vi "HW5p1_Task1_Solution (2).vi"() -> ()   [LabVIEW 2016]
panel:
  out "D (nC/cm^2)":dbl
  in  "r (cm)":dbl
  in  "rho_v (nC/cm^3)":dbl
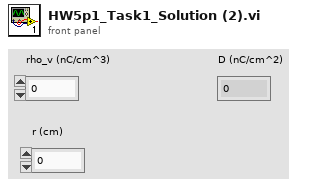
[diagram p1: front panel]
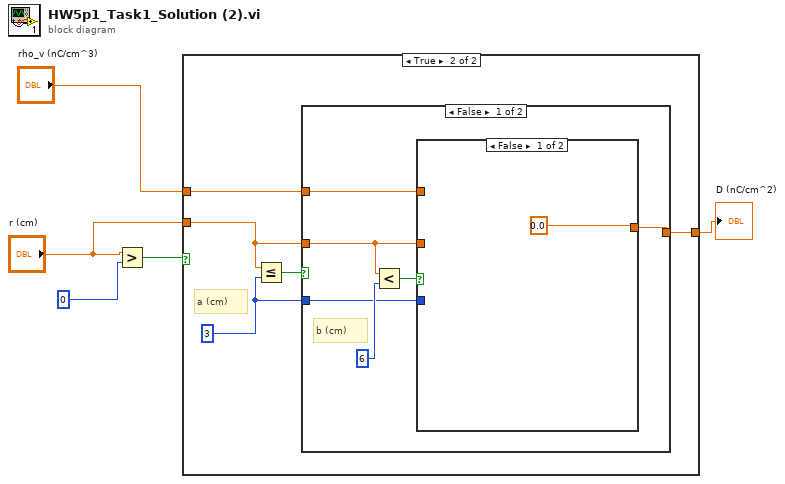
[diagram p0: block diagram]
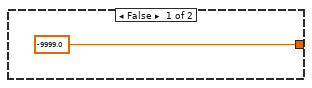
[diagram p2: hidden frame]
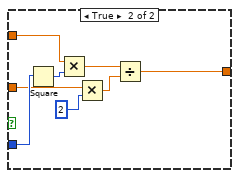
[diagram p3: hidden frame]
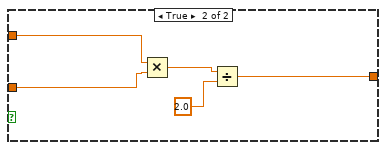
[diagram p4: hidden frame]
diagram:
  n1 = Greater?(x="r (cm)", y=0) -> (0:w5:bool)
  n2 = case shown="True" w5 {
    tunnel: "r (cm)" -> [_ w9]
    tunnel: "rho_v (nC/cm^3)" -> [_ w10]
    tunnel: [-9999.0 w8] -> w1
    frame False {
    }
    frame True {
      w7 = 3
      # "a (cm)"
      n3 = Less Or Equal?(x=w9, y=w7) -> (x <= y?=w11:bool)
      n4 = case shown="False" w11 {
        tunnel: w10 -> [w15 w31]
        tunnel: w9 -> [w13 w30]
        tunnel: [w12 w27] -> w8
        tunnel: w7 -> [w14 _]
        frame False {
          # "b (cm)"
          n5 = Less?(x=w13, y=6) -> (x < y?=w17:bool)
          n6 = case shown="False" w17 {
            tunnel: w15 -> [_ w26]
            tunnel: w14 -> [_ w24]
            tunnel: w13 -> [_ w20]
            tunnel: [0.0 w19] -> w12
            frame False {
            }
            frame True {
              n7 = Square(x=w24) -> (x^2=w25:i32)
              n8 = Multiply(x=w26, y=w25) -> (x*y=w23:dbl)
              n9 = Multiply(x=w20, y=2) -> (x*y=w22:dbl)
              n10 = Divide(x=w23, y=w22) -> (x/y=w19:dbl)
            }
          }
        }
        frame True {
          n11 = Multiply(x=w31, y=w30) -> (x*y=w29:dbl)
          n12 = Divide(x=w29, y=2.0) -> (x/y=w27:dbl)
        }
      }
    }
  }
  "D (nC/cm^2)" <- w1
